vi "Log VNA Data Test.vi"() -> ()   [LabVIEW 2023]
uses:
  LibreVNA/Types/Trace Enum.ctl
  LibreVNA/LibreVNA.lvclass
panel:
  out "size(s)":i32[](array[numeric])
  out "XY Graph":cluster{"Array":dbl[], "Array":dbl[]}(graph)
  in  "Trace Name":T1
  out "FileSaved":bool
  in  "LogStartTime":timestamp
  in  "PartName":string
  in  "Path in":path=path "C:/Projects/Data"
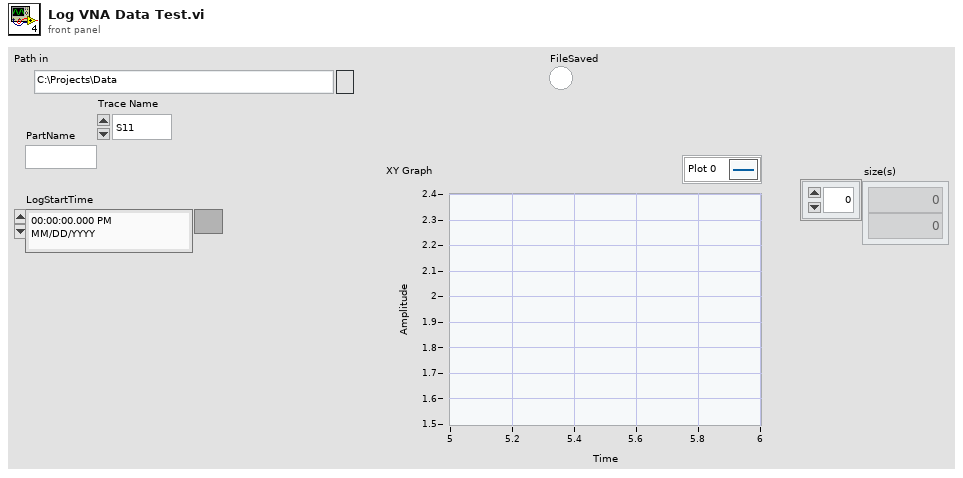
[diagram p1: front panel]
types:
  T1 = typedef "LibreVNA.lvclass/Trace Enum.ctl" = enum16{"S11", "S12", "S21", "S22"}
  T2 = typedef "UI Data.ctl" = cluster{"session":refnum<class "Modbus Master.lvclass">, "IsOpen":bool, "Timeout (ms)":i32, "TempFile":path, "LogStartTime":timestamp, "LibreVNA":refnum<class "LibreVNA.lvclass">, "VNAOpen":bool, "TempSP":dbl, "ActualTemp":dbl, "FileSaved":bool, "PIDOutput":dbl, "VNALogOpt":refnum<vi>, "PartName":string, "ComPort":refnum<visa-resource-name>, "S-Param Data":dbl[][], "VNADataFile":path}
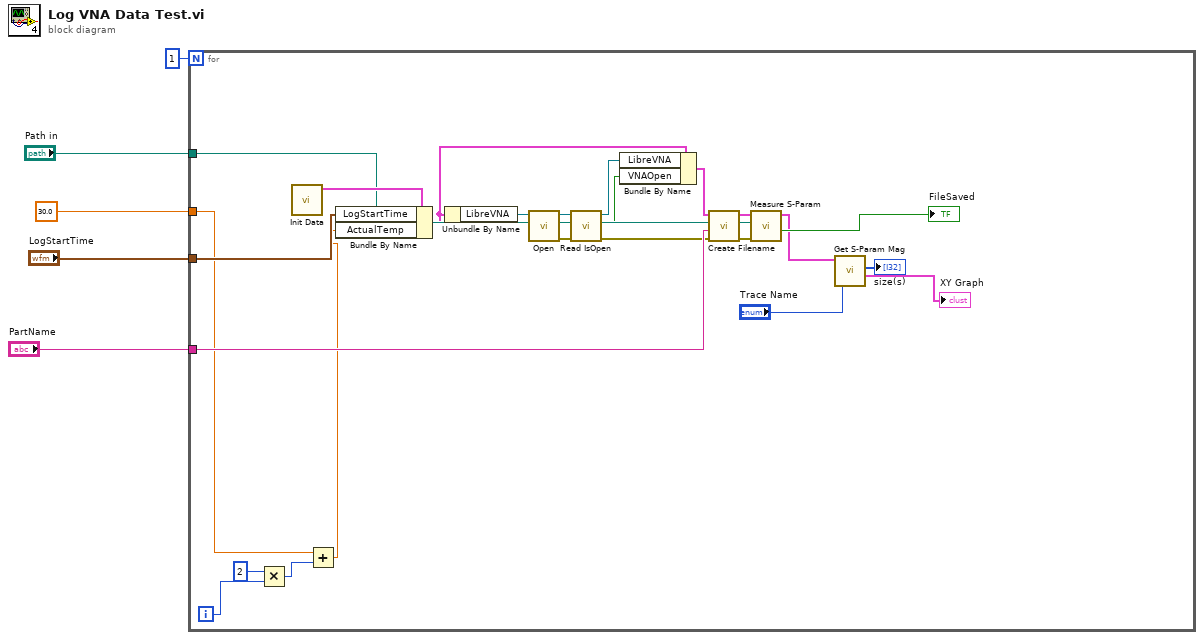
[diagram p0: block diagram]
diagram:
  n1 = for {
    N: 1 -> [_]
    tunnel: "Path in" -> [w29]
    tunnel: "PartName" -> [w28]
    tunnel: "LogStartTime" -> [w24]
    tunnel: 30.0 ("ActualTemp") -> [w7]
    i -> [w10]
    n2 = Multiply(x=2, y=w10) -> (x*y=w8:i32)
    n3 = call "Init Data.vi"() -> ("Data Out"=w30:T2)  [unwired: 11 in]
    n4 = Add(x=w7, y=w8) -> (x+y=w6:dbl)
    n5 = Bundle By Name(cluster=w30, "LogStartTime"=w24, "ActualTemp"=w6) -> (w22:T2)
    n6 = Unbundle By Name(w22) -> ("LibreVNA"=w21:refnum<class "LibreVNA.lvclass">)
    n7 = call-dynamic "Open.vi"("LibreVNA in"=w21) -> ("error out"=w19:errorcluster, "LibreVNA out"=w20:refnum<class "LibreVNA.lvclass">)  [unwired: 9 in]
    n8 = call-dynamic "Read IsOpen.vi"("error in (no error)"=w19, "LibreVNA in"=w20) -> ("error out"=w15:errorcluster, "IsOpen"=w16:bool, "LibreVNA out"=w17:refnum<class "LibreVNA.lvclass">)  [unwired: 7 in]
    n9 = Bundle By Name(cluster=w22, "LibreVNA"=w17, "VNAOpen"=w16) -> (w18:T2)
    n10 = call "Create Filename.vi"("error in"=w15, "PartName"=w28, "Path in"=w29, "Data in"=w18) -> ("error out"=w25:errorcluster, "FileName"=w26:path, "Data Out"=w27:T2)  [unwired: 5 in]
    n11 = call "Measure S-Param.vi"("error in (no error)"=w25, "DataFile"=w26, "Data in"=w27) -> ("FileSaved"=→"FileSaved":bool, "Data Out out"=w14:T2)  [unwired: 2 in, 1 out]
    n12 = call "Get S-Param Mag.vi"("Trace Name"="Trace Name", "Data in"=w14) -> ("Graph"=→"XY Graph":cluster{"Array":dbl[], "Array":dbl[]}, "size(s)"=→"size(s)":i32[])  [unwired: 2 in, 2 out]
  }
